vi "Invert Tank Drive.vi"(2 "Toggle":bool, 3 "Value 2":dbl, 4 "Value 1":dbl) -> (0 "Value 2":dbl, 1 "Value 1":dbl)   [LabVIEW 2015]
uses:
  <vilib>/Rock Robotics/Network Tables/NT Write Boolean.vi
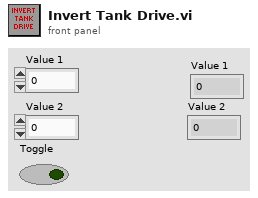
[diagram p1: front panel]
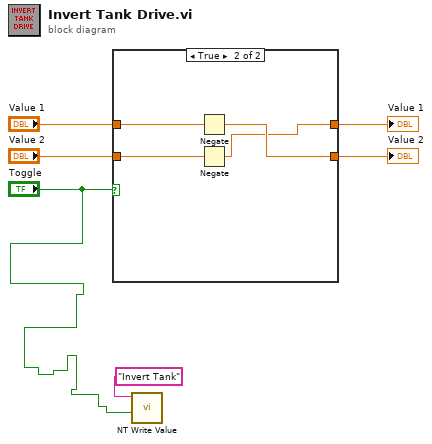
[diagram p0: block diagram]
diagram:
  n1 = case shown="True" "Toggle" {
    tunnel: "Value 1" -> [w8 w12]
    tunnel: "Value 2" -> [w7 w11]
    tunnel: [w7 w10] -> w4
    tunnel: [w8 w9] -> w3
    frame False {
    }
    frame True {
      n2 = Negate(x=w12) -> (-x=w10:dbl)
      n3 = Negate(x=w11) -> (-x=w9:dbl)
    }
  }
  "Value 2" <- w4
  "Value 1" <- w3
  n4 = call-poly <vilib>:"NT Write Value.vi"("Boolean"="Toggle", "Name"="Invert Tank") -> ()  [unwired: 9 in, 1 out]
